vi "ChequeaDatos.vi"() -> ()   [LabVIEW 2010]
panel:
  out "Signals":dynamicdata(graph)=[{"t0"=timestamp(0 s since 1904-01-01), "dt"=1.0, "Y"=array[1018 elements], "attributes"=variant("NI_ChannelName"=variant(string "u"), "NI_ExpIsRelativeTime"=variant(bool TRUE), "NI_ExpStartTimeStamp"=variant(timestamp timestamp(3323044175.96875 s since 1904-01-01)), "NI_ExpTimeStamp"=variant(timestamp timestamp(3323044175.96875 s since 1904-01-01)), "NI_ExpXDimension"=variant(string "t"))}, {"t0"=timestamp(0 s since 1904-01-01), "dt"=1.0, "Y"=array[1018 elements], "attributes"=variant("NI_ChannelName"=variant(string "Temp"), "NI_ExpIsRelativeTime"=variant(bool TRUE), "NI_ExpStartTimeStamp"=variant(timestamp timestamp(3323044175.96875 s since 1904-01-01)), "NI_ExpTimeStamp"=variant(timestamp timestamp(3323044175.96875 s since 1904-01-01)), "NI_ExpXDimension"=variant(string "t"))}]
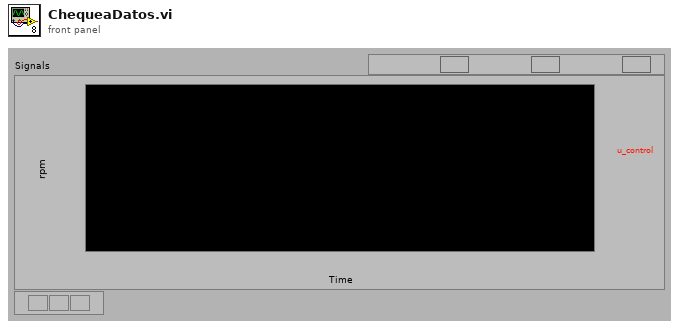
[diagram p1: front panel]
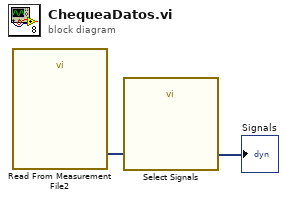
[diagram p0: block diagram]
diagram:
  n1 = call "Read From Measurement File2"() -> ("Signals"=w2:dynamicdata)  [unwired: 6 in, 5 out]
  n2 = call "Select Signals"("Signals"=w2) -> ("Signal Out"=→"Signals":dynamicdata)  [unwired: 2 in, 8 out]
